vi "Get last image.vi"(8 "error in (no error)":errorcluster, 11 "IMAQdx Cam in":refnum<class "IMAQdx Cam.lvclass">) -> (0 "error out":errorcluster, 2 "Image Out":T1, 3 "IMAQdx Cam out":refnum<class "IMAQdx Cam.lvclass">)   [LabVIEW 2020, in "IMAQdx Cam.lvclass"]
uses:
  IMAQdx Cam.lvclass
  <vilib>/vision/Image Controls.llb/IMAQ Image.ctl
  <vilib>/vision/driver/IMAQdx.llb/IMAQdx Buffer Number Mode.ctl
  IMAQdx Cam.lvclass/IMAQdx Cam.ctl
  <vilib>/vision/driver/NI_Vision_Acquisition_Software.lvlib
  <vilib>/vision/NI_Vision_Development_Module.lvlib
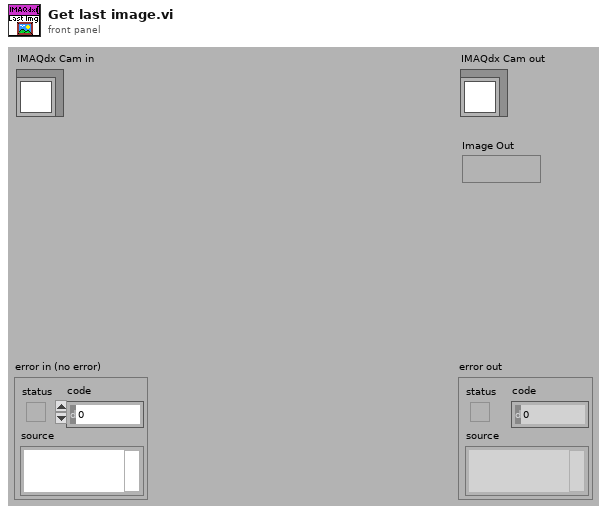
[diagram p1: front panel]
types:
  T1 = typedef "IMAQ Image.ctl" = refnum<image>
  T2 = typedef "NI_Vision_Acquisition_Software.lvlib/IMAQdx Buffer Number Mode.ctl" = enum32{"Next", "Last", "Buffer Number", "Every", "Last New"}
  T3 = typedef "IMAQdx.ctl" = refnum<k21>
  T4 = typedef "Image Type" = u32
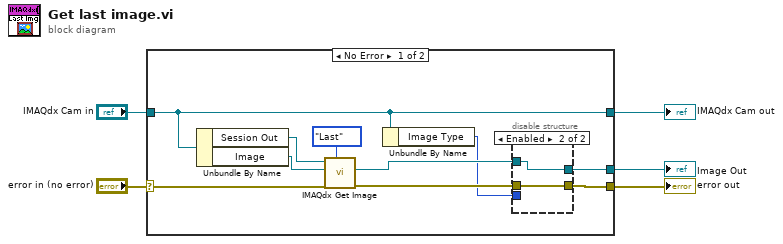
[diagram p0: block diagram]
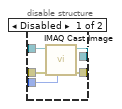
[diagram p2: hidden frame]
diagram:
  n1 = case shown="No Error" "error in (no error)" {
    selector: "error in (no error)" -> [w13 w24]
    tunnel: [w10 w24] -> w2
    tunnel: [w7 w23] -> w3
    tunnel: "IMAQdx Cam in" -> [w7 w23]
    tunnel: [w8 _] -> w1
    frame No Error {
      n2 = Unbundle By Name(w7) -> ("Session Out"=w14:T3, "Image"=w12:T1)
      n3 = call <vilib>:"IMAQdx Get Image.vi"("Buffer Number Mode (Next)"=IMAQdx_Buffer_Number_Mode."Last" ("Buffer Number Mode"), "error in"=w13, "Image In"=w12, "Session In"=w14) -> ("error out"=w11:errorcluster, "Image Out"=w9:T1)  [unwired: 1 in, 5 out]
      n4 = Unbundle By Name(w7) -> ("Image Type"=w6:T4)
      n5 = disable-structure shown="Enabled" {
        disable-tunnel: w11 -> [w20 w21]
        disable-tunnel: [w19 w21] -> w10
        disable-tunnel: w9 -> [w18 w22]
        disable-tunnel: [w17 w22] -> w8
        disable-tunnel: w6 -> [w16 _]
        frame Disabled {
          n6 = call "IMAQ Cast Image"("Image Type"=w16, "error in (no error)"=w20, "Image Src"=w18) -> ("error out"=w19:errorcluster, "Image Dst Out"=w17:T1)  [unwired: 7 in]
        }
        frame Enabled {
        }
      }
    }
    frame Error {
    }
  }
  "error out" <- w2
  "IMAQdx Cam out" <- w3
  "Image Out" <- w1
